vi "DataFromDB.vi"(8 "error in":errorcluster, 9 "all string":string, 10 "Procedure name":string, 11 "DSN name":string) -> (0 "error out":errorcluster caption="错误输出", 1 "DataOut":string[][](array[string]), 3 "Result":string)   [LabVIEW 2013]
uses:
  <vilib>/addons/database/Connection.llb/DB Tools Open Connec (String).vi
  <vilib>/addons/database/Connection.llb/Conn Execute.vi
  <vilib>/addons/database/Recordset.llb/Rec Fetch Recordset Data (R).vi
  <vilib>/addons/database/Recordset.llb/Rec Destroy - Connection.vi
  <vilib>/addons/database/NI_Database_API.lvlib
panel:
  out "连接的字符串":string
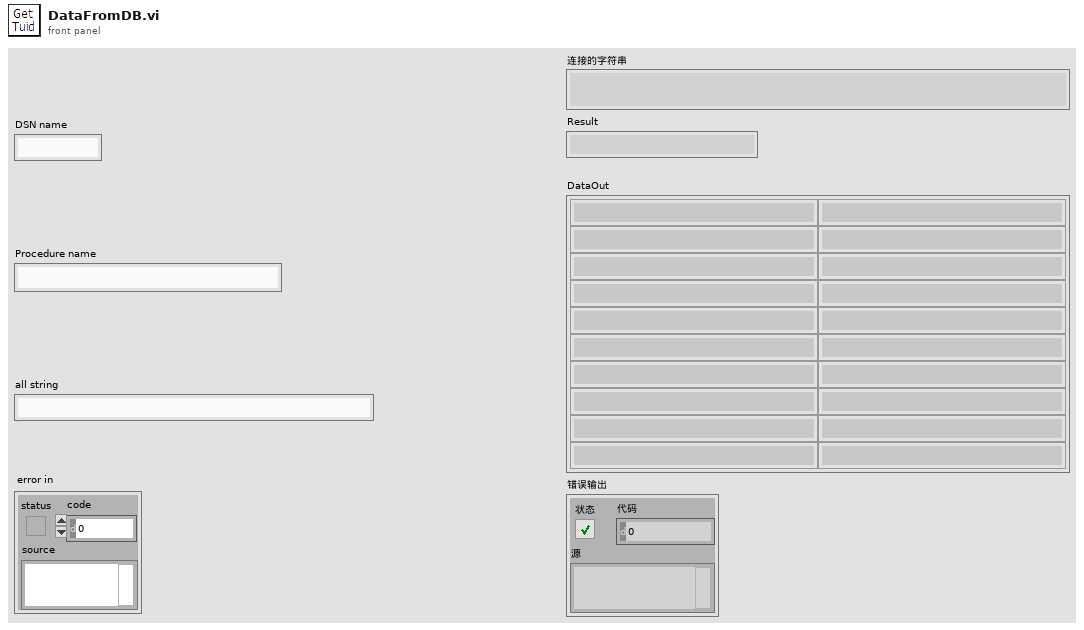
[diagram p1: front panel]
types:
  T1 = typedef "NI_Database_API.lvlib/Conn ObjectReference.ctl" = refnum<k1>
  T2 = typedef "NI_Database_API.lvlib/Rec ObjectReference.ctl" = refnum<k1>
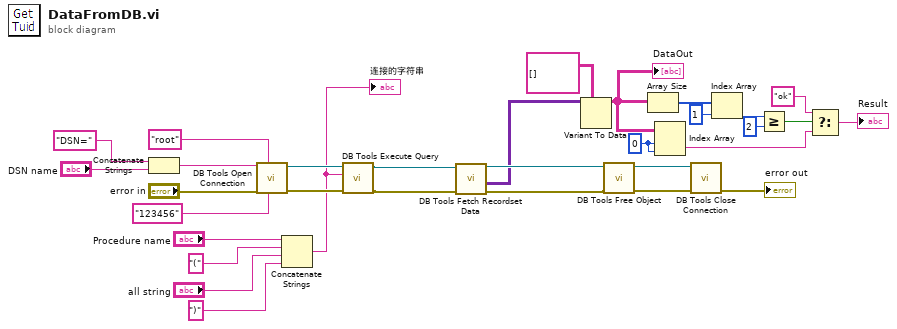
[diagram p0: block diagram]
diagram:
  w4 = 0 ("索引")
  n1 = Concatenate Strings("DSN=", "DSN name") -> (w22:string)
  n2 = call-poly <vilib>:"DB Tools Open Connection.vi"("password"="123456" ("userID"), "userID"="root", "error in (no error)"="error in", "connection information"=w22) -> ("error out"=w32:errorcluster, "connection reference"=w31:T1)  [unwired: 4 in]
  n3 = Concatenate Strings("Procedure name", "(", "all string", ")") -> (w27:string)
  "连接的字符串" <- w27
  n4 = call-poly <vilib>:"DB Tools Execute Query.vi"("error in (no error)"=w32, "SQL query"=w27, "connection reference"=w31) -> ("error out"=w16:errorcluster, "recordset reference"=w17:T2)  [unwired: 5 in]
  n5 = call-poly <vilib>:"DB Tools Fetch Recordset Data.vi"("error in (no error)"=w16, "recordset reference"=w17) -> ("error out"=w14:errorcluster, "recordset data"=w12:variant[][], "recordset reference out"=w15:T2)  [unwired: 3 in]
  n6 = Variant To Data(type=string[][] [], Variant=w12) -> (data=w5:string[][])  [unwired: 1 in, 1 out]
  "DataOut" <- w5
  n7 = call-poly <vilib>:"DB Tools Free Object.vi"("error in (no error)"=w14, "recordset reference"=w15) -> ("error out"=w29:errorcluster, "connection reference"=w30:T1)  [unwired: 8 in]
  n8 = Array Size(array=w5) -> (size(s)=w11:i32[])
  n9 = Index Array(array=w5, index (row)=w4, index (col)=w4) -> (element=w3:string)
  n10 = call <vilib>:"DB Tools Close Connection.vi"("error in (no error)"=w29, "connection reference"=w30) -> ("error out"=→"error out":errorcluster)  [unwired: 5 in]
  n11 = Index Array(array=w11, index=1 ("索引")) -> (element=w9:i32)
  n12 = Greater Or Equal?(x=w9, y=2) -> (x >= y?=w7:bool)
  n13 = Select(t="ok", s=w7, f=w3) -> (s? t:f=→"Result":string)
